vi "Close Starter Kit.vi"(8 "error in (no error)":errorcluster, 11 "starter kit host in":refnum<class "NI_Robotics_Starter Kit Host.lvclass">) -> (0 "error out":errorcluster)   [LabVIEW 2017, in "NI_Robotics_Starter Kit Host.lvclass"]
doc: "<B>Owning Palette:</B> Starter Kit 1.0 VIs, Starter Kit 2.0 VIs\n\nTerminates a communication session with the FPGA on a real or simulated Starter Kit robot. When the communication session ends, the drive motors, distance sensor, and sensor servo stop operating."
uses:
  <vilib>/robotics/Starter Kit/Host Interface/NI_Robotics_Starter Kit Host.lvclass
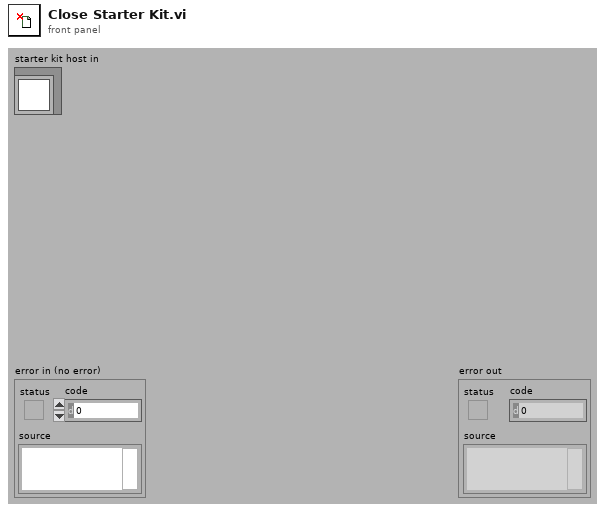
[diagram p1: front panel]
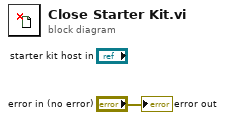
[diagram p0: block diagram]
diagram:
  "error out" <- "error in (no error)"
